vi "DSF.Common.Constants.vi"   [LabVIEW 2016, in "DSF.Common.lvlib"]
uses:
  DSF.Common.lvlib
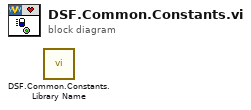
[diagram p0: block diagram]
diagram:
  n1 = call "DSF.Common.Constants.Library Name.vi"() -> ()  [unwired: 11 in, 1 out]
